vi "S2C_VLFT10_Proc_GetExtCommStatus.vi"(7 "Timeout":dbl, 8 "Error In":errorcluster, 11 "Status":string) -> (0 "Error Out":errorcluster, 3 "Result":string)   [LabVIEW 2015]
uses:
  Fornax/VIs/PolyDriver/Typedefs/ExternalCommPairingStatus.ctl
  Fornax/VIs/PolyDriver/Typedefs/DftMode.ctl
  Fornax/VIs/S2C_FORNAX_Proc_Globals.vi
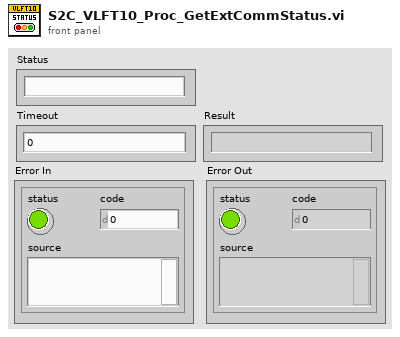
[diagram p1: front panel]
types:
  T1 = cluster{"PostDelay (ms)":i32, "ClearFornaxMsgs":bool}
  T2 = typedef "ExternalCommPairingStatus.ctl" = i16
  T3 = typedef "DftMode.ctl" = i16
  T4 = cluster{"Partition":string, "Message":string, "M_ControllerBoardId":string, "M_ChassisSerialNumber":string, "M_Alias":string, "M_PrimaryIpAddress":string, "M_PairingStatus":T2, "M_PairedEntityIpAddress":string, "M_PairedEntityAlias":string, "M_PairedEntityId":string, "M_Options":string, "M_DftMode":T3, "M_IsViperEnabled":bool, "M_Crc32":i32}
  T5 = cluster{"Partition":string, "Message":string, "M_ControllerBoardId":string, "M_ChassisSerialNumber":string, "M_Alias":string, "M_PrimaryIpAddress":string, "M_PairingStatus":T2, "M_PairedEntityIpAddress":string, "M_PairedEntityAlias":string, "M_PairedEntityId":string, "M_Options":string, "M_DftMode":T3, "M_IsViperEnabled":bool}
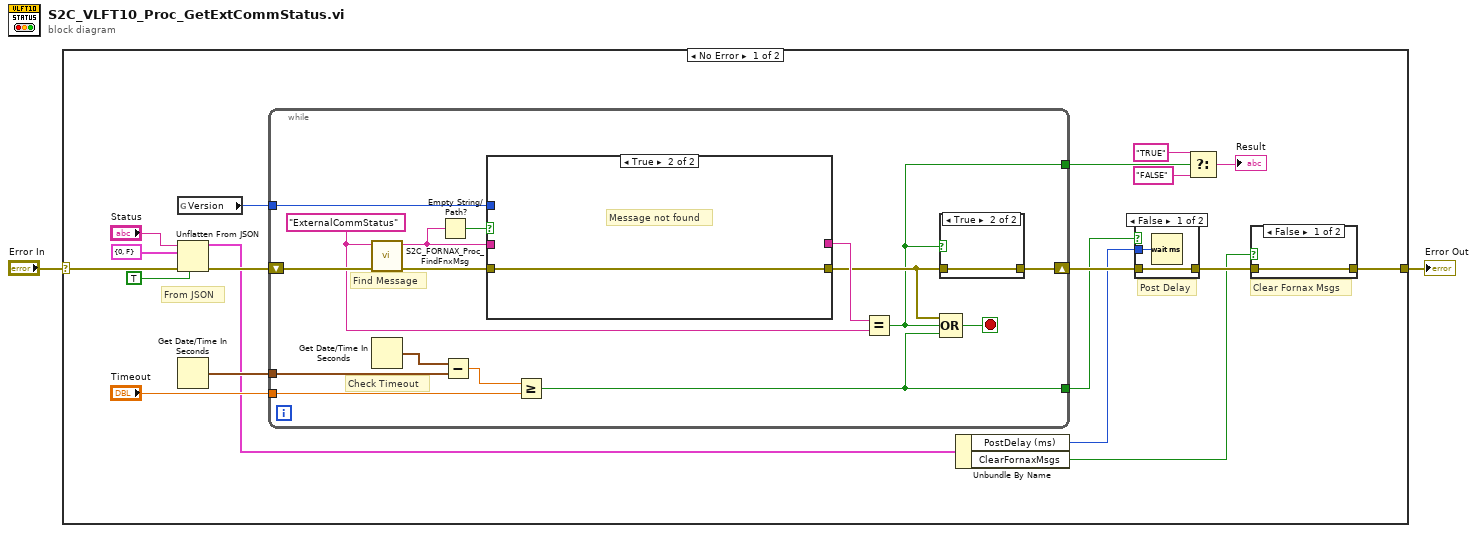
[diagram p0: block diagram]
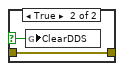
[diagram p2: hidden frame]
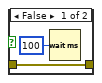
[diagram p4: hidden frame]
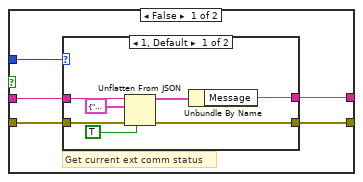
[diagram p5: hidden frame]
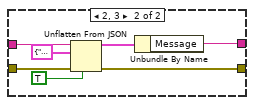
[diagram p6: hidden frame]
diagram:
  n1 = case shown="No Error" "Error In" {
    selector: "Error In" -> [w18 w67]
    tunnel: [w9 w67] -> w1
    frame No Error {
      # "Clear Fornax Msgs"
      # "Post Delay"
      # "From JSON"
      n2 = global read "S2C_FORNAX_Proc_Globals.vi" "Version"() -> (w21:i32)
      n3 = Unflatten From JSON(JSON string="Status", type and defaults=T1 {"PostDelay (ms)"=0, "ClearFornaxMsgs"=FALSE}, default null elements? (F)=TRUE, error in (no error)=w18) -> (value=w14:T1, error out=w17:errorcluster)  [unwired: 3 in]
      n4 = Get Date/Time In Seconds() -> (seconds since 1Jan1904=w16:timestamp)
      n5 = while {
        tunnel: w21 -> [w42]
        shift-right: [w31] -> w13
        shift-left: w17 -> [w41]
        tunnel: w16 -> [w37]
        tunnel: "Timeout" -> [w36]
        tunnel: [w30] -> w12
        tunnel: [w28] -> w6
        stop <- w34 stop-if-true
        w29 = "ExternalCommStatus" ("MsgName")
        # "Check Timeout"
        # "Find Message"
        n6 = call "S2C_FORNAX_Proc_FindFnxMsg.vi"("Error In"=w41, "MsgName"=w29) -> ("Error Out"=w43:errorcluster, "Message"=w39:string)  [unwired: 8 in]
        n7 = Get Date/Time In Seconds() -> (seconds since 1Jan1904=w38:timestamp)
        n8 = Empty String/Path?(string/path=w39) -> (empty?=w40:bool)
        n9 = Subtract(x=w38, y=w37) -> (x-y=w35:dbl)
        n10 = case shown="True" w40 {
          tunnel: w43 -> [w51 w66]
          tunnel: w42 -> [w50 _]
          tunnel: [w49 w66] -> w32
          tunnel: [w48 _] -> w33
          tunnel: w39 -> [w47 _]
          frame False {
            # "Get current ext comm status"
            n11 = case shown="1, Default" w50 {
              tunnel: w51 -> [w57 w64]
              tunnel: [w55 w62] -> w49
              tunnel: [w54 w61] -> w48
              tunnel: w47 -> [w53 w60]
              frame 1, Default {
                n12 = Unflatten From JSON(JSON string=w53, type and defaults=T4 {"Partition"="", "Message"="", "M_ControllerBoardId"="", "M_ChassisSerialNumber"="", "M_Alias"="", "M_PrimaryIpAddress"="", "M_PairingStatus"=3, "M_PairedEntityIpAddress"="", "M_PairedEntityAlias"="", "M_PairedEntityId"="", "M_Options"="", "M_DftMode"=0, "M_IsViperEnabled"=TRUE, "M_Crc32"=0}, default null elements? (F)=TRUE, error in (no error)=w57) -> (value=w56:T4, error out=w55:errorcluster)  [unwired: 3 in]
                n13 = Unbundle By Name(w56) -> ("Message"=w54:string)
              }
              frame 2, 3 {
                n14 = Unflatten From JSON(JSON string=w60, type and defaults=T5 {"Partition"="", "Message"="", "M_ControllerBoardId"="", "M_ChassisSerialNumber"="", "M_Alias"="", "M_PrimaryIpAddress"="", "M_PairingStatus"=3, "M_PairedEntityIpAddress"="", "M_PairedEntityAlias"="", "M_PairedEntityId"="", "M_Options"="", "M_DftMode"=0, "M_IsViperEnabled"=TRUE}, default null elements? (F)=TRUE, error in (no error)=w64) -> (value=w63:T5, error out=w62:errorcluster)  [unwired: 3 in]
                n15 = Unbundle By Name(w63) -> ("Message"=w61:string)
              }
            }
          }
          frame True {
            # "Message not found"
          }
        }
        n16 = Greater Or Equal?(x=w35, y=w36) -> (x >= y?=w30:bool)
        n17 = Equal?(x=w33, y=w29) -> (x = y?=w28:bool)
        n18 = case shown="True" w28 {
          tunnel: w32 -> [w45 w46]
          tunnel: [w45 w46] -> w31
          frame False {
            n19 = Wait (ms)(milliseconds to wait=u32 100) -> ()  [unwired: 1 out]
          }
          frame True {
          }
        }
        n20 = Compound Arithmetic op=OR(w32, w28, w30) -> (w34:bool)
      }
      n21 = Unbundle By Name(w14) -> ("PostDelay (ms)"=w11:i32, "ClearFornaxMsgs"=w8:bool)
      n22 = case shown="False" w12 {
        tunnel: w13 -> [w26 w27]
        tunnel: [w26 w27] -> w10
        tunnel: w11 -> [w25 _]
        frame False {
          n23 = Wait (ms)(milliseconds to wait=w25) -> ()  [unwired: 1 out]
        }
        frame True {
        }
      }
      n24 = Select(t="TRUE", s=w6, f="FALSE") -> (s? t:f=→"Result":string)
      n25 = case shown="False" w8 {
        selector: w8 -> [_ w23]
        tunnel: w10 -> [w22 w24]
        tunnel: [w22 w24] -> w9
        frame False {
        }
        frame True {
          n26 = global write "S2C_FORNAX_Proc_Globals.vi" "ClearDDS"(w23) -> ()
        }
      }
    }
    frame Error {
    }
  }
  "Error Out" <- w1
